vi "QTrkAccurateTickCount.vi"() -> (0 "seconds":dbl, 1 "tick count (ms)":dbl)   [LabVIEW 2011]
uses:
  kernel32.dll
panel:
  out "freq":u64
  out "count":u64
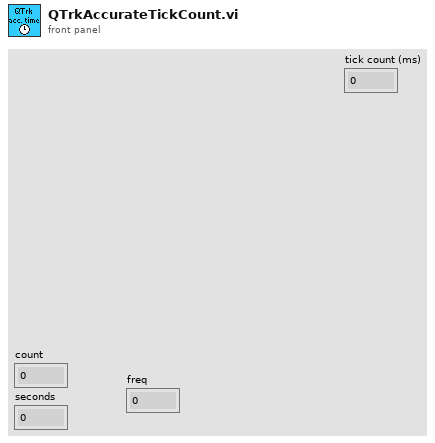
[diagram p1: front panel]
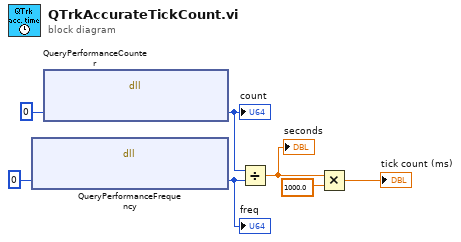
[diagram p0: block diagram]
diagram:
  n1 = dll-call lib="kernel32.dll" fn="QueryPerformanceFrequency"("frequency"=u64 0) -> ("frequency"=w5:u64)  [unwired: 4 in, 2 out]
  "freq" <- w5
  n2 = dll-call lib="kernel32.dll" fn="QueryPerformanceCounter"("counter"=u64 0) -> ("counter"=w4:u64)  [unwired: 4 in, 2 out]
  "count" <- w4
  n3 = Divide(x=w4, y=w5) -> (x/y=w3:dbl)
  "seconds" <- w3
  n4 = Multiply(x=w3, y=1000.0) -> (x*y=→"tick count (ms)":dbl)
